vi "PH_HamamatsuCamera.set Numeric Cam Attribute Tip Strip.vi"(1 "Minimum":dbl, 2 "Maximum":dbl, 3 "Attribute":string) -> (0 "Tip Strip":string)   [LabVIEW 2014, in "PH_HamamatsuCamera.lvlib"]
doc: "This VI sets a numeric Cam Attribute tip strip."
uses:
  PH_HamamatsuCamera.lvlib
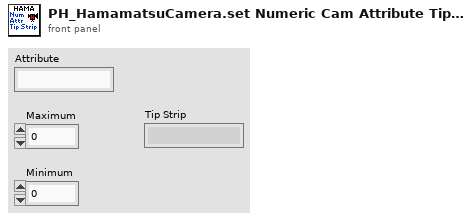
[diagram p1: front panel]
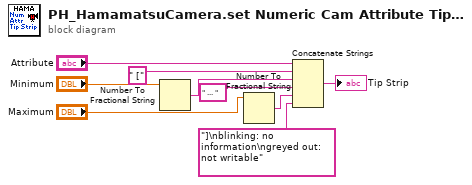
[diagram p0: block diagram]
diagram:
  n1 = Number To Fractional String(number="Minimum") -> (F-format string=w5:string)  [unwired: 3 in]
  n2 = Number To Fractional String(number="Maximum") -> (F-format string=w6:string)  [unwired: 3 in]
  n3 = Concatenate Strings("Attribute", " [" ("string"), w5, " ... " ("string"), w6, "]\nblinking: no information\ngreyed out: not writable") -> (→"Tip Strip":string)
